vi "readPress.vi"() -> ()   [LabVIEW 2015]
uses:
  <vilib>/Utility/file.llb/Read From Spreadsheet File (string).vi
panel:
  out "today file":string
  out "Pressure":string[][](table)
  in  "EXIT":bool
  in  "OK Button":bool
  in  "Boolean":bool caption="Choose date    Today"
  out "Pressure":cluster{dbl[], dbl[]}[](graph)=[{[1.0, 2.0, 4.0], [2.0, 1.0, 0.0]}, {[0.5, 1.5, 3.5], [3.0, 4.0, 2.0]}]
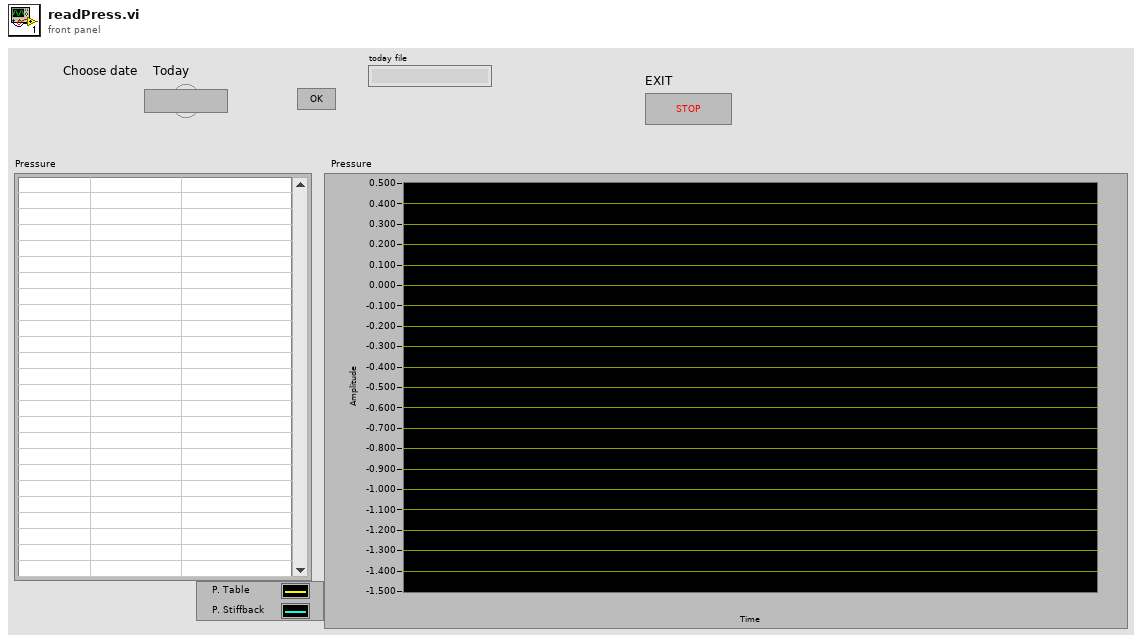
[diagram p1: front panel]
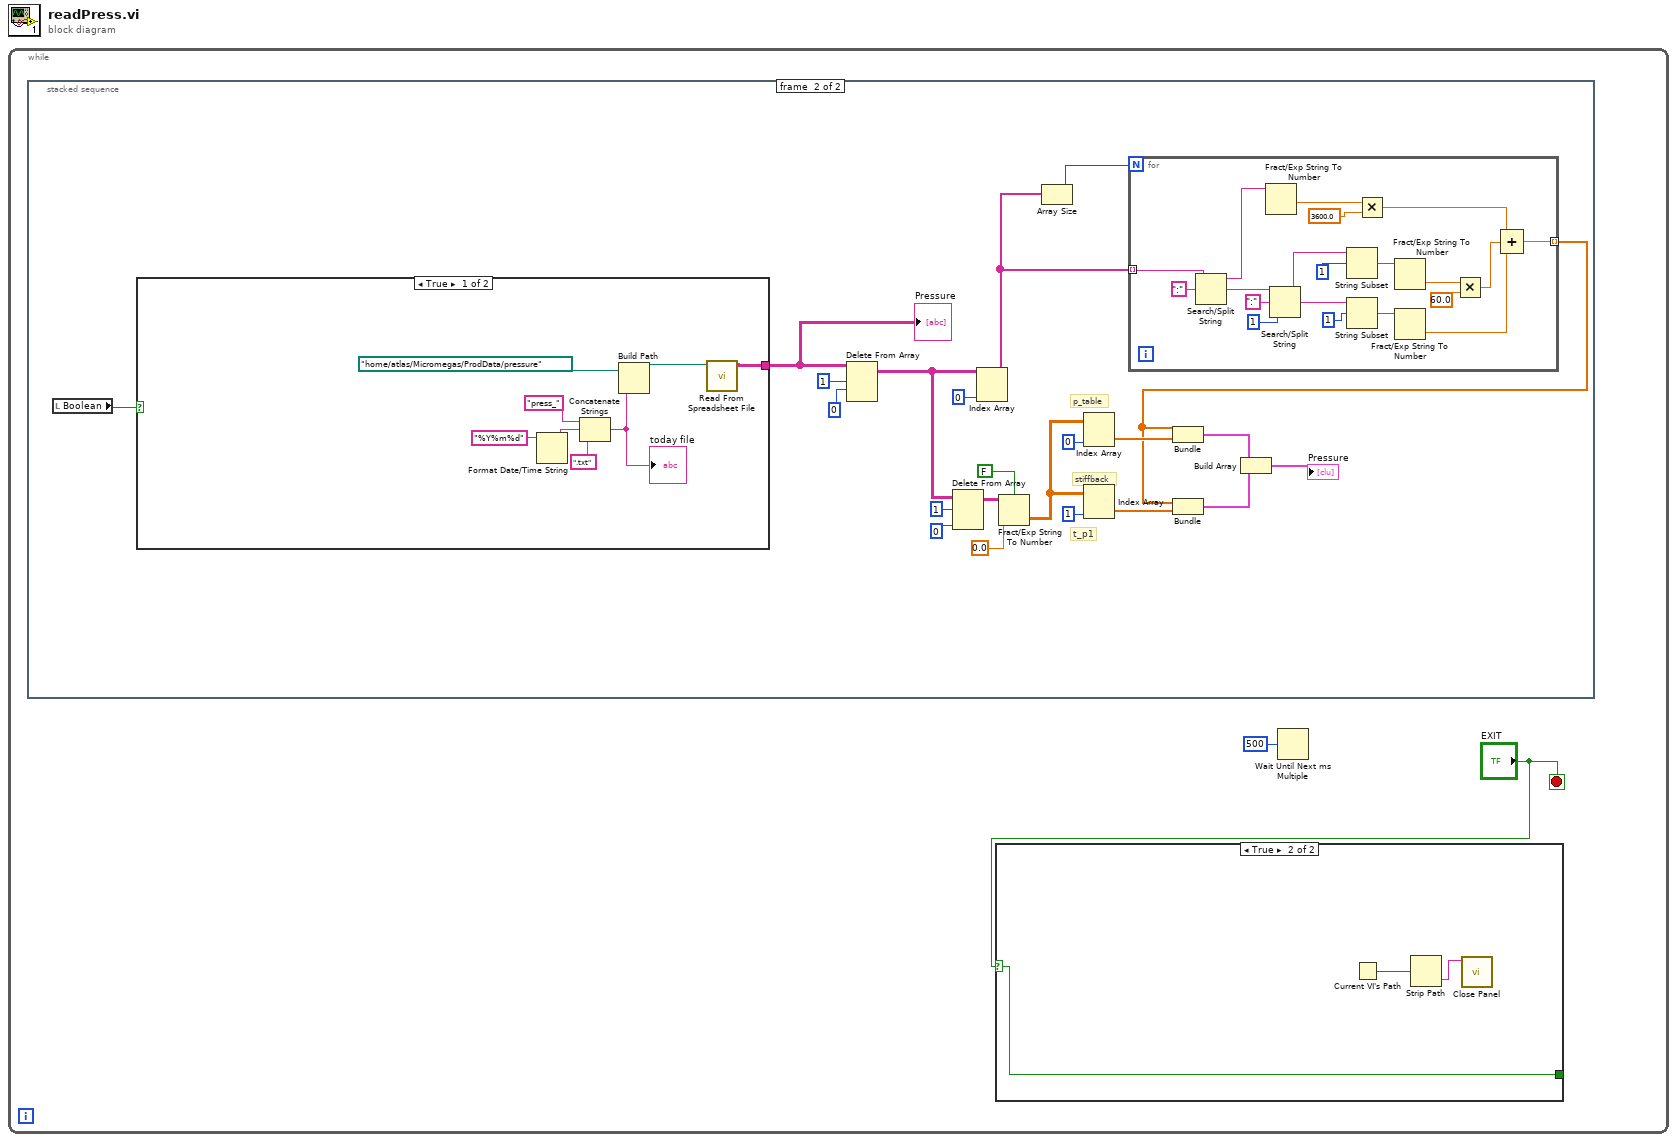
[diagram p0: block diagram]
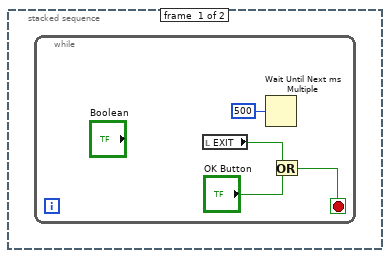
[diagram p3: hidden frame]
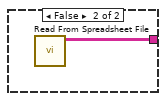
[diagram p4: hidden frame]
diagram:
  n1 = while {
    stop <- "EXIT" stop-if-true
    n2 = stacked-sequence {
      frame #0 {
        n3 = while {
          stop <- w7 stop-if-true
          n4 = local read "EXIT"() -> (w9:bool)
          n5 = Wait Until Next ms Multiple(millisecond multiple=u32 500) -> ()  [unwired: 1 out]
          n6 = Or(x=w9, y="OK Button") -> (x .or. y?=w7:bool)
        }
      }
      frame #1 {
        # "t_p1"
        # "stiffback"
        # "p_table"
        n7 = local read "Boolean"() -> (w13:bool)
        n8 = case shown="True" w13 {
          tunnel: [w35 w41] -> w11
          frame True {
            n9 = Format Date/Time String(time format string (%c)="%Y%m%d") -> (date/time string=w38:string)  [unwired: 2 in]
            n10 = Concatenate Strings("press_" ("string"), w38, ".txt" ("string")) -> (w36:string)
            "today file" <- w36
            n11 = Build Path(base path=path "/home/atlas/Micromegas/ProdData/pressure", name or relative path=w36) -> (appended path=w33:path)
            n12 = call-poly <vilib>:"Read From Spreadsheet File.vi"("file path (dialog if empty)"=w33) -> ("all rows"=w35:string[][])  [unwired: 6 in, 4 out]
          }
          frame False {
            n13 = call-poly <vilib>:"Read From Spreadsheet File.vi"() -> ("all rows"=w41:string[][])  [unwired: 7 in, 4 out]
          }
        }
        "Pressure" <- w11
        n14 = Delete From Array(array=w11, length=1, index (row)=0) -> (array with subset deleted=w12:string[][])  [unwired: 1 in, 1 out]
        n15 = Delete From Array(array=w12, length=1, index (col)=0 ("disabled index (col)")) -> (array with subset deleted=w29:string[][])  [unwired: 1 in, 1 out]
        n16 = Index Array(array=w12, index (col)=0 ("disabled index (col)")) -> (element=w27:string[])  [unwired: 1 in]
        n17 = Fract/Exp String To Number(use system decimal point (T)=FALSE, string=w29, default (0 dbl)=0.0 ("default (0 DBL)")) -> (number=w18:dbl[][])  [unwired: 1 in, 1 out]
        n18 = Array Size(array=w27) -> (size(s)=w28:i32)
        n19 = Index Array(array=w18, index (col)=0 ("disabled index (col)")) -> (element=w22:dbl[])  [unwired: 1 in]
        n20 = Index Array(array=w18, index (col)=1 ("disabled index (col)")) -> (element=w21:dbl[])  [unwired: 1 in]
        n21 = for {
          N: w28 -> [_]
          tunnel: w27 -> [w61] mode=indexing
          tunnel: [w53] -> w17 mode=indexing
          n22 = Search/Split String(string=w61, search string/char (-)=":") -> (substring before match=w57:string, match + rest of string=w58:string)  [unwired: 1 in, 1 out]
          n23 = Fract/Exp String To Number(string=w57) -> (number=w45:dbl)  [unwired: 3 in, 1 out]
          n24 = Search/Split String(string=w58, search string/char (-)=":", offset (0)=1) -> (substring before match=w51:string, match + rest of string=w47:string)  [unwired: 1 out]
          n25 = String Subset(string=w51, offset (0)=1) -> (substring=w49:string)  [unwired: 1 in]
          n26 = String Subset(string=w47, offset (0)=1) -> (substring=w46:string)  [unwired: 1 in]
          n27 = Multiply(x=w45, y=3600.0) -> (x*y=w44:dbl)
          n28 = Fract/Exp String To Number(string=w49) -> (number=w54:dbl)  [unwired: 3 in, 1 out]
          n29 = Fract/Exp String To Number(string=w46) -> (number=w42:dbl)  [unwired: 3 in, 1 out]
          n30 = Multiply(x=w54, y=60.0) -> (x*y=w43:dbl)
          n31 = Compound Arithmetic op=ADD(w44, w43, w42) -> (w53:dbl)
        }
        n32 = Bundle(w17, w22) -> (w16:cluster{dbl[], dbl[]})  [unwired: 1 in]
        n33 = Bundle(w17, w21) -> (w15:cluster{dbl[], dbl[]})  [unwired: 1 in]
        n34 = Build Array(w16, w15) -> (→"Pressure":cluster{dbl[], dbl[]}[])
      }
    }
    n35 = case shown="True" "EXIT" {
      selector: "EXIT" -> [w3 w6]
      tunnel: [w3 w6] -> _
      frame False {
      }
      frame True {
        n36 = Current VI's Path() -> (path=w4:path)
        n37 = Strip Path(path=w4) -> (name=w5:string)  [unwired: 1 out]
        n38 = call <vilib>:"Close Panel.vi"("VI name"=w5) -> ()  [unwired: 10 in, 1 out]
      }
    }
    n39 = Wait Until Next ms Multiple(millisecond multiple=u32 500) -> ()  [unwired: 1 out]
  }
